vi "MenuShortcut_Globals.vi"() -> ()   [LabVIEW 2016]
panel:
  in  "whitespace text":string[][](array[string])=[[" ", "空格"], ["\t", "制表符"]] caption="空白字符文本"
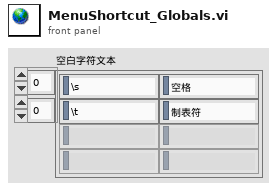
[diagram p1: front panel]
diagram:
